vi "StartExperiment.vi"(11 "Experiment In":T1={"File Path"=path "", "Operator"="", "Project"="", "Target Dose (dpa)"=0.0, "Sample"={"Name"="", "Description"="", "Molar Mass (g/mol)"=0.0, "Density (g/cm^3)"=0.0, "Irradiation Area (cm^2)"=0.0, "SRIM Damage Peak (disp * ions/cm)"=0.0}, "Beam Line"={"Type"=enum."Ion Beam Analysis", "Ion"=enum."H", "Charge State"=0, "Total Source Ion Energy (kV)"=nan}, "Runs"=[]} {"Beam Line"."Charge State" min=1}) -> (2 "Experiment Run":T6, 3 "Experiment Out":T1={"File Path"=path "", "Operator"="", "Project"="", "Target Dose (dpa)"=0.0, "Sample"={"Name"="", "Description"="", "Molar Mass (g/mol)"=0.0, "Density (g/cm^3)"=0.0, "Irradiation Area (cm^2)"=0.0, "SRIM Damage Peak (disp * ions/cm)"=0.0}, "Beam Line"={"Type"=enum."Ion Beam Analysis", "Ion"=enum."H", "Charge State"=0, "Total Source Ion Energy (kV)"=nan}, "Runs"=[]} {"Beam Line"."Charge State" min=1})   [LabVIEW 2012]
uses:
  Experiment.ctl
  Sample.ctl
  BeamLine.ctl
  BeamLineType.ctl
  BeamLineIon.ctl
  ExperimentRun.ctl
  ExperimentRunTiming.ctl
  ExperimentRunDose.ctl
  ExperimentRunFluence.ctl
  ExperimentRunTotalCharge.ctl
panel:
  out "Start Fluence (ions/cm^2)":dbl
  out "Start Dose (dpa)":dbl
  out "Start Current (A)":dbl
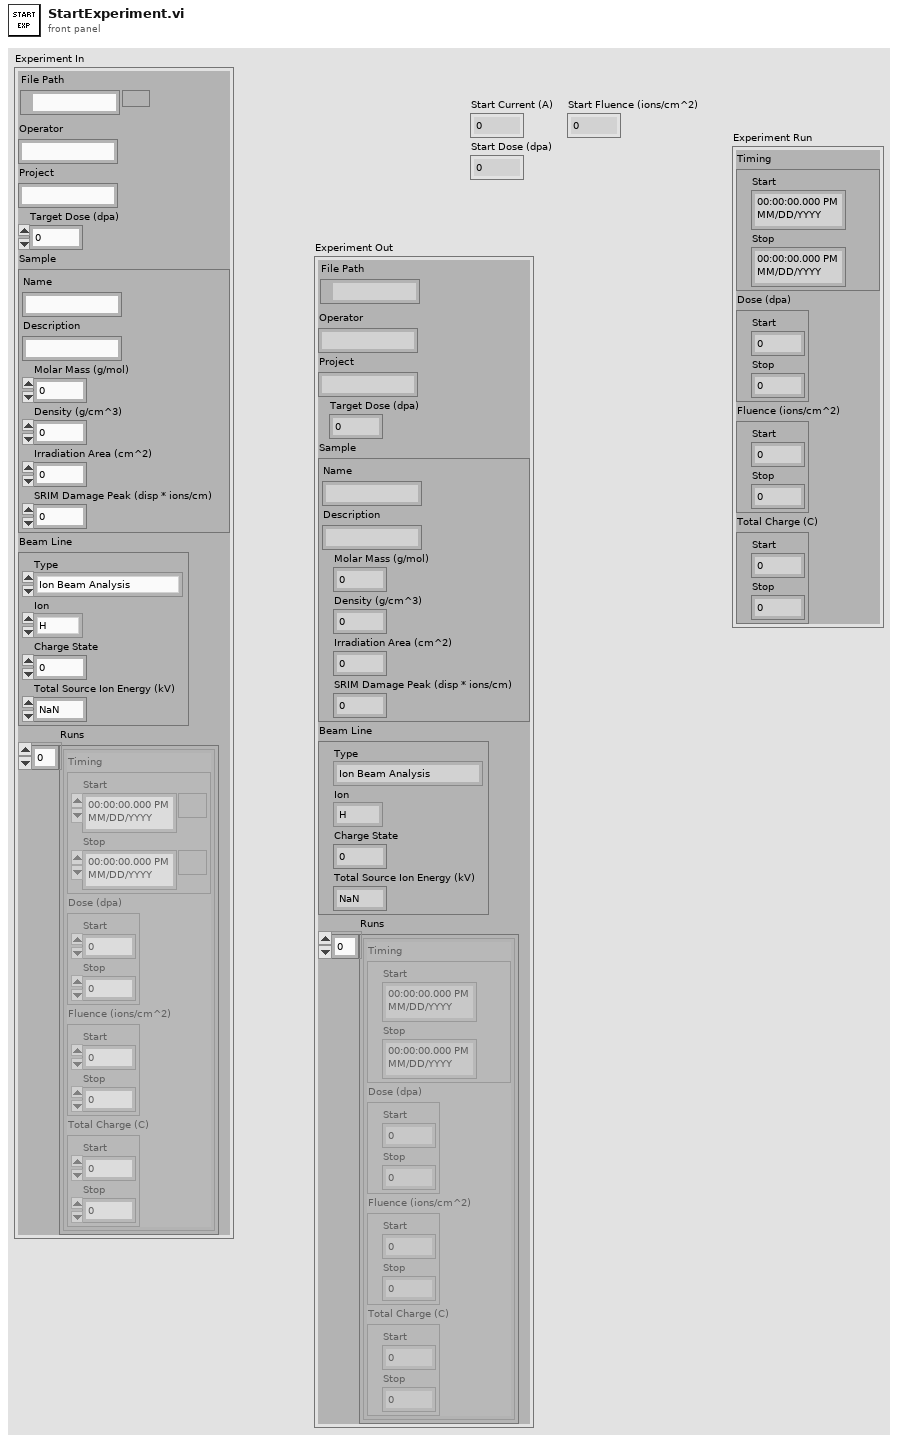
[diagram p1: front panel]
types:
  T1 = typedef "Experiment.ctl" = cluster{"File Path":path, "Operator":string, "Project":string, "Target Dose (dpa)":dbl, "Sample":T2, "Beam Line":T3, "Runs":T6[]}
  T2 = typedef "Sample.ctl" = cluster{"Name":string, "Description":string, "Molar Mass (g/mol)":dbl, "Density (g/cm^3)":dbl, "Irradiation Area (cm^2)":dbl, "SRIM Damage Peak (disp * ions/cm)":dbl}
  T3 = typedef "BeamLine.ctl" = cluster{"Type":T4, "Ion":T5, "Charge State":u8, "Total Source Ion Energy (kV)":dbl}
  T4 = typedef "BeamLineType.ctl" = enum16{"Ion Beam Analysis", "Auxiliary", "Radiation Damage"}
  T5 = typedef "BeamLineIon.ctl" = enum16{"H", "He", "C", "Fe", "Ni", "Pt", "Si", "Ag", "Au"}
  T6 = typedef "ExperimentRun.ctl" = cluster{"Timing":T7, "Dose (dpa)":T8, "Fluence (ions/cm^2)":T9, "Total Charge (C)":T10}
  T7 = typedef "ExperimentRunTiming.ctl" = cluster{"Start":timestamp, "Stop":timestamp}
  T8 = typedef "ExperimentRunDose.ctl" = cluster{"Start":dbl, "Stop":dbl}
  T9 = typedef "ExperimentRunFluence.ctl" = cluster{"Start":dbl, "Stop":dbl}
  T10 = typedef "ExperimentRunTotalCharge.ctl" = cluster{"Start":dbl, "Stop":dbl}
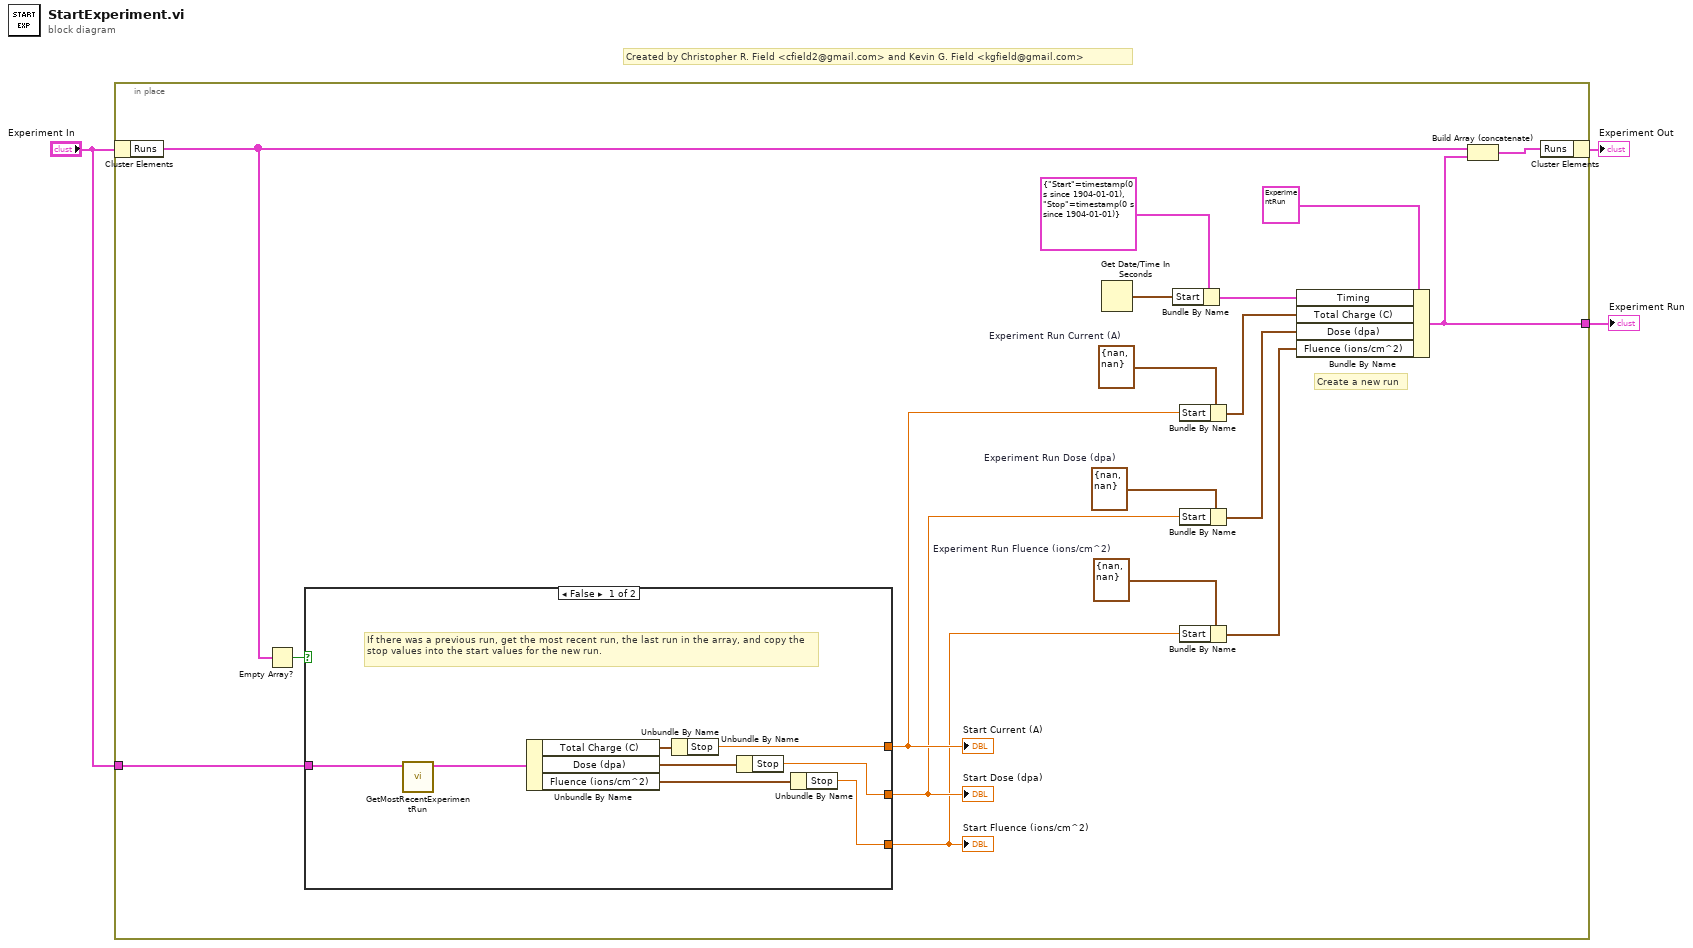
[diagram p0: block diagram]
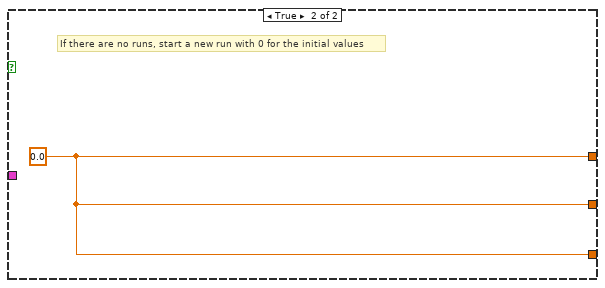
[diagram p2: hidden frame]
diagram:
  # "Created by Christopher R. Field <cfield2@gmail.com> and Kevin G. Field <kgfield@gmail.com>"
  n1 = in-place {
    in-place-border: [w5] -> w2
    in-place-border: "Experiment In" -> [w4]
    w16 = T10 {"Start"=nan, "Stop"=nan}  # Experiment Run Current (A)
    w15 = T9 {"Start"=nan, "Stop"=nan}  # Experiment Run Fluence (ions/cm^2)
    w17 = T8 {"Start"=nan, "Stop"=nan}  # Experiment Run Dose (dpa)
    # "Create a new run"
    n2 = in-place-cluster #1("Experiment In") -> ("Runs"=w7:T6[])
    n3 = Empty Array?(array=w7) -> (empty?=w21:bool)
    n4 = case shown="False" w21 {
      tunnel: [w22 w30] -> w12
      tunnel: [w23 w30] -> w13
      tunnel: [w24 w30] -> w14
      tunnel: w4 -> [w29 _]
      frame False {
        # "If there was a previous run, get the most recent run, the last run in the array, and copy the stop values into the start values for the new run."
        n5 = call "GetMostRecentExperimentRun.vi"("Experiment"=w29) -> ("Recent Experiment Run"=w28:T6)  [unwired: 10 in]
        n6 = Unbundle By Name(w28) -> ("Total Charge (C)"=w27:T10, "Dose (dpa)"=w26:T8, "Fluence (ions/cm^2)"=w25:T9)
        n7 = Unbundle By Name(w27) -> ("Stop"=w24:dbl)
        n8 = Unbundle By Name(w26) -> ("Stop"=w23:dbl)
        n9 = Unbundle By Name(w25) -> ("Stop"=w22:dbl)
      }
      frame True {
        w30 = 0.0 ("Stop")
        # "If there are no runs, start a new run with 0 for the initial values"
      }
    }
    "Start Current (A)" <- w14
    "Start Dose (dpa)" <- w13
    "Start Fluence (ions/cm^2)" <- w12
    n10 = Get Date/Time In Seconds() -> (seconds since 1Jan1904=w18:timestamp)
    n11 = Bundle By Name(cluster=T7 {"Start"=timestamp(0 s since 1904-01-01), "Stop"=timestamp(0 s since 1904-01-01)} ("Experiment Run Timing"), "Start"=w18) -> (w11:T7)
    n12 = Bundle By Name(cluster=w16, "Start"=w14) -> (w10:T10)
    n13 = Bundle By Name(cluster=w17, "Start"=w13) -> (w9:T8)
    n14 = Bundle By Name(cluster=w15, "Start"=w12) -> (w8:T9)
    n15 = Bundle By Name(cluster=T6 {"Timing"={"Start"=timestamp(0 s since 1904-01-01), "Stop"=timestamp(0 s since 1904-01-01)}, "Dose (dpa)"={"Start"=0.0, "Stop"=0.0}, "Fluence (ions/cm^2)"={"Start"=0.0, "Stop"=0.0}, "Total Charge (C)"={"Start"=0.0, "Stop"=0.0}} ("Experiment Run"), "Timing"=w11, "Total Charge (C)"=w10, "Dose (dpa)"=w9, "Fluence (ions/cm^2)"=w8) -> (w5:T6)
    n16 = Build Array (concatenate)(w7, w5) -> (w6:T6[])
    n17 = in-place-cluster #1("Runs"=w6) -> (→"Experiment Out":T1)
  }
  "Experiment Run" <- w2
